vi "tcs_getSample_kernelSite.vi"(8 "error in (no error)":errorcluster, 11 "kernel_Site_Ctl":T1={"Amprms[21]"=[0.0, 0.0, 0.0, 0.0, 0.0, 0.0, 0.0, 0.0, 0.0, 0.0, 0.0, 0.0, 0.0, 0.0, 0.0, 0.0, 0.0, 0.0, 0.0, 0.0, 0.0], "Aoprms[15]"=[0.0, 0.0, 0.0, 0.0, 0.0, 0.0, 0.0, 0.0, 0.0, 0.0, 0.0, 0.0, 0.0, 0.0, 0.0], "Daz"=0.0, "Diurab"=0.0, "Elong"=0.0, "Lat"=0.0, "Refa"=0.0, "Refb"=0.0, "St0"=0.0, "T0"=0.0, "Tt0"=0.0, "Ttj"=0.0, "Ttmtai"=0.0, "Uau"=0.0, "Ukm"=0.0, "Vau"=0.0, "Vkm"=0.0, "delat"=0.0, "delut"=0.0, "elongm"=0.0, "hm"=0.0, "latm"=0.0, "tai"=0.0, "ttmtat"=0.0, "xpm"=0.0, "ypm"=0.0}) -> (0 "error out":errorcluster, 2 "function return":i32, 3 "kernel_Site_Ctl out":T1)   [LabVIEW 2016, in "SALLV_tcs.lvlib"]
doc: "int tcs_shm_getSample_kernel_SiteLV(tcs_kernel_SiteLV *kernel_Site_Ctl );"
uses:
  SALLV_tcs.lvlib
  DataTypes/kernel_Site.ctl
  SALLV_tcs.so
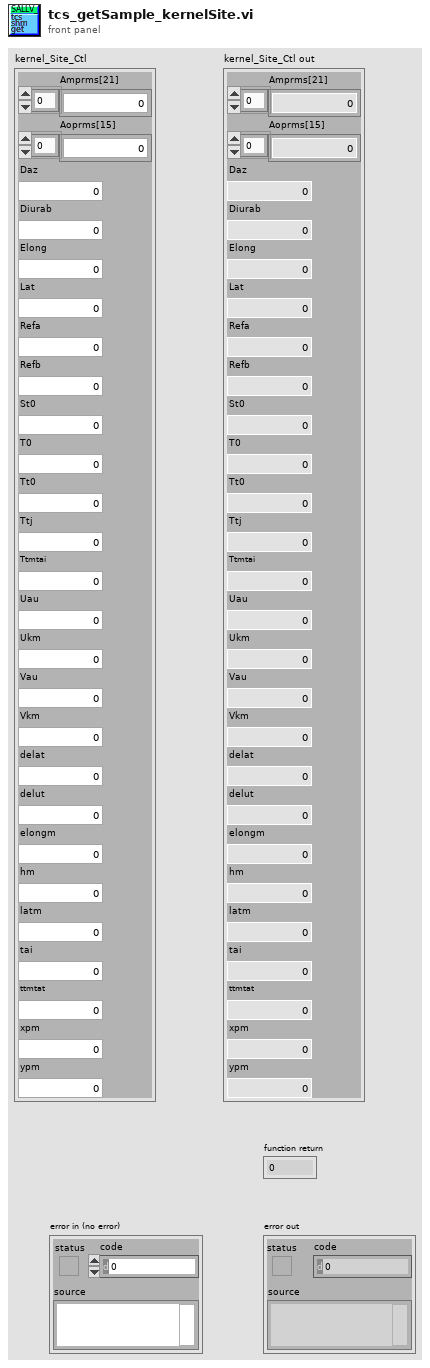
[diagram p1: front panel]
types:
  T1 = typedef "SALLV_tcs.lvlib/kernel_Site.ctl" = cluster{"Amprms[21]":sgl[], "Aoprms[15]":sgl[], "Daz":sgl, "Diurab":sgl, "Elong":sgl, "Lat":sgl, "Refa":sgl, "Refb":sgl, "St0":sgl, "T0":sgl, "Tt0":sgl, "Ttj":sgl, "Ttmtai":sgl, "Uau":sgl, "Ukm":sgl, "Vau":sgl, "Vkm":sgl, "delat":sgl, "delut":sgl, "elongm":sgl, "hm":sgl, "latm":sgl, "tai":sgl, "ttmtat":sgl, "xpm":sgl, "ypm":sgl}
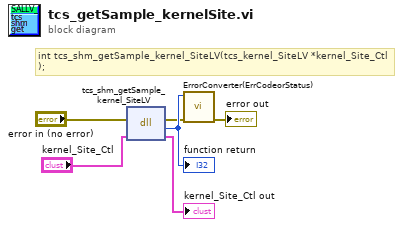
[diagram p0: block diagram]
diagram:
  # "int tcs_shm_getSample_kernel_SiteLV(tcs_kernel_SiteLV *kernel_Site_Ctl );"
  n1 = dll-call lib="home/andres/Desktop/SALLV_tcs/SALLV_tcs.*" fn="tcs_shm_getSample_kernel_SiteLV"(error in="error in (no error)", "kernel_Site_Ctl"="kernel_Site_Ctl") -> (error out=w2:errorcluster, w6:i32, "kernel_Site_Ctl"=→"kernel_Site_Ctl out":T1)  [unwired: 2 in, 1 out]
  "function return" <- w6
  n2 = call "ErrorConverter(ErrCodeorStatus).vi"("error in (no error)"=w2, "error code"=w6) -> ("error out"=→"error out":errorcluster)  [unwired: 9 in]
